vi "MonofasicSimluator.vi"() -> ()   [LabVIEW 2011]
panel:
  out "S":cdb
  out "XY Graph":cluster{"X":dbl[], "Y":dbl[]}[](graph)
  out "Amplitud\nVoltaje":dbl
  out "Amplitud\nCorriente":dbl
  in  "Phase":dbl
  out "Señales\nTemporales":dynamicdata(graph) caption="Sine"
  out "Diagrama Fasorial":picture
  out "Q":dbl
  out "P":dbl
  out "I":dbl
  # "El angulo representa la impedancia\nde las señales"
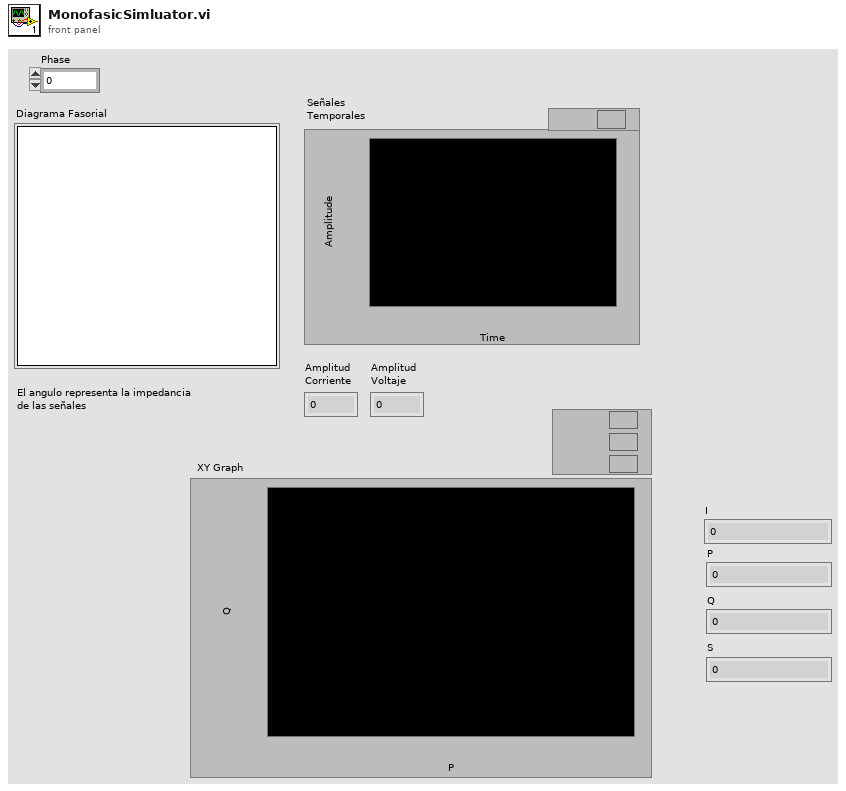
[diagram p1: front panel]
types:
  T1 = typedef "LVBoundsTypeDef.ctl" = cluster{"Width":u32, "Height":u32}
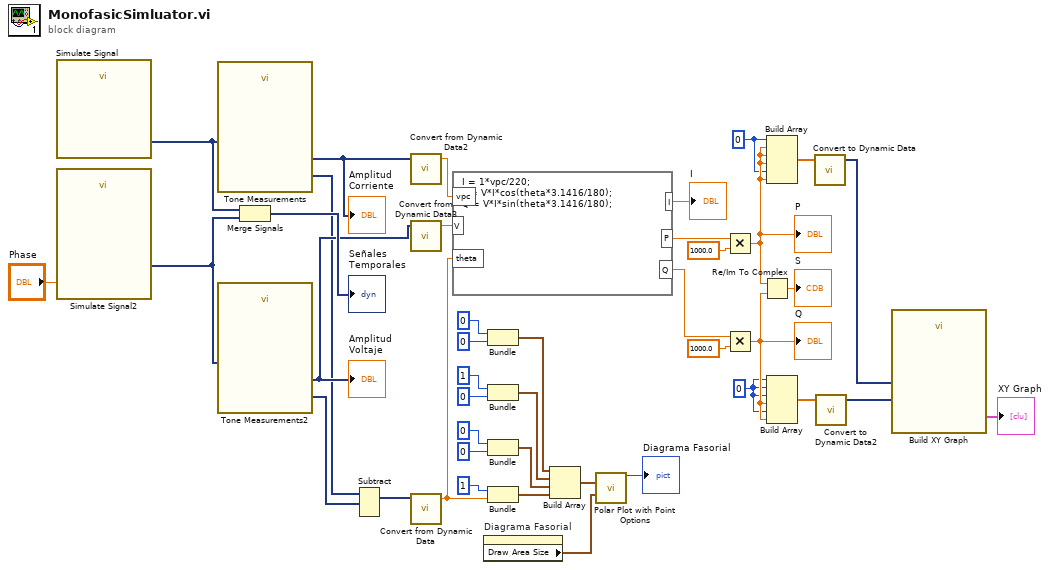
[diagram p0: block diagram]
diagram:
  w1 = 0
  w2 = 0
  n1 = call "Simulate Signal"() -> ("Sine"=w20:dynamicdata)  [unwired: 14 in, 1 out]
  n2 = call "Simulate Signal2"("Phase"="Phase") -> ("Sine"=w19:dynamicdata)  [unwired: 13 in, 1 out]
  n3 = call "Tone Measurements"("Signals"=w20) -> ("Phase"=w11:dynamicdata, "Amplitude"=w16:dynamicdata)  [unwired: 7 in, 2 out]
  "Amplitud\nCorriente" <- w16
  n4 = call "Tone Measurements2"("Signals"=w19) -> ("Phase"=w10:dynamicdata, "Amplitude"=w15:dynamicdata)  [unwired: 7 in, 2 out]
  "Amplitud\nVoltaje" <- w15
  n5 = Merge Signals(w20, w19) -> (→"Señales\nTemporales":dynamicdata)
  n6 = Subtract(1:w10, 2:w11) -> (0:w18:dynamicdata)  [unwired: 1 in, 1 out]
  n7 = call "Convert from Dynamic Data2"("Dynamic Data Type"=w16) -> ("Scalar"=w14:dbl)  [unwired: 3 in]
  n8 = call "Convert from Dynamic Data3"("Dynamic Data Type"=w15) -> ("Scalar"=w13:dbl)  [unwired: 3 in]
  n9 = call "Convert from Dynamic Data"("Dynamic Data Type"=w18) -> ("Scalar"=w17:dbl)  [unwired: 3 in]
  n10 = formula code="I = 1*vpc/220;\nP = V*I*cos(theta*3.1416/180);\nQ = V*I*sin(theta*3.1416/180);"("vpc"=w14, "theta"=w17, "V"=w13) -> ("I"=→"I":dbl, "P"=w40:dbl, "Q"=w39:dbl)
  n11 = property on="Diagrama Fasorial" class="Pict"() -> ("Draw Area Size"=w36:T1)  [unwired: 2 in, 2 out]
  n12 = Bundle(0, 0) -> (w30:cluster{i32, i32})  [unwired: 1 in]
  n13 = Bundle(1, 0) -> (w29:cluster{i32, i32})  [unwired: 1 in]
  n14 = Bundle(0, 0) -> (w25:cluster{i32, i32})  [unwired: 1 in]
  n15 = Bundle(1, "Scalar"=w17) -> (w22:cluster{i32, "Scalar":dbl})  [unwired: 1 in]
  n16 = Build Array(w30, w29, w25, w22) -> (w28:cluster{i32, "Scalar":dbl}[])
  n17 = call <vilib>:"Polar Plot with Point Options.vi"("data array [mag, phase (deg)]"=w28, "dimensions (w,h)"=w36) -> ("new picture"=→"Diagrama Fasorial":picture)  [unwired: 13 in]
  n18 = Multiply(x=w40, y=1000.0) -> (x*y=w6:dbl)
  "P" <- w6
  n19 = Multiply(x=w39, y=1000.0) -> (x*y=w5:dbl)
  "Q" <- w5
  n20 = Re/Im To Complex(1:w5, 2:w6) -> (0:→"S":cdb)
  n21 = Build Array(w2, w6, w6, w6, w2, w6) -> (w8:dbl[])
  n22 = Build Array(w1, w1, w1, w5, w1, w5) -> (w4:dbl[])
  n23 = call "Convert to Dynamic Data"("Array"=w8) -> ("Dynamic Data Type"=w7:dynamicdata)  [unwired: 3 in]
  n24 = call "Convert to Dynamic Data2"("Array"=w4) -> ("Dynamic Data Type"=w3:dynamicdata)  [unwired: 3 in]
  n25 = call "Build XY Graph"("Y Input"=w3, "X Input"=w7) -> ("XY Graph"=→"XY Graph":cluster{"X":dbl[], "Y":dbl[]}[])  [unwired: 8 in, 1 out]
